vi "Configure Frequency.vi"(0 "VISA resource name":refnum<visa-resource-name>, 5 "Frequency Mode (0: Fixed)":i32(ring) items=["Fixed", "Step", "Pulse", "List", "Sense", "External"], 7 "Frequency (60 Hz)":dbl=60.0, 9 "Triggered Frequency (60 Hz)":dbl=60.0, 11 "error in (no error)":errorcluster) -> (4 "VISA resource name out":refnum<visa-resource-name>, 15 "error out":errorcluster)   [LabVIEW 2013, in "California Instruments iX Series.lvlib"]
doc: "Configures the output frequency of the AC source."
uses:
  California Instruments iX Series.lvlib
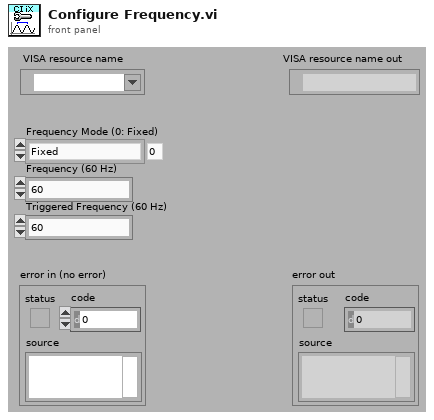
[diagram p1: front panel]
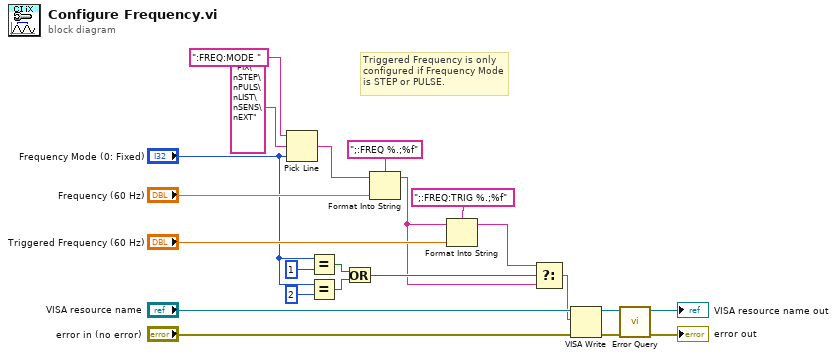
[diagram p0: block diagram]
diagram:
  # "Triggered Frequency is only configured if Frequency Mode is STEP or PULSE."
  n1 = Pick Line(string ("")=":FREQ:MODE ", multi-line string="FIX\nSTEP\nPULS\nLIST\nSENS\nEXT", line index="Frequency Mode (0: Fixed)") -> (output string=w14:string)
  n2 = Equal?(x="Frequency Mode (0: Fixed)", y=1) -> (x = y?=w6:bool)
  n3 = Equal?(x="Frequency Mode (0: Fixed)", y=2) -> (x = y?=w5:bool)
  n4 = Or(x=w6, y=w5) -> (x .or. y?=w4:bool)
  n5 = Format Into String(format string=";:FREQ %.;%f", initial string=w14, "Frequency (60 Hz)") -> (resulting string=w2:string)  [unwired: 1 in, 1 out]
  n6 = Format Into String(format string=";:FREQ:TRIG %.;%f", initial string=w2, "Triggered Frequency (60 Hz)") -> (resulting string=w1:string)  [unwired: 1 in, 1 out]
  n7 = Select(t=w1, s=w4, f=w2) -> (s? t:f=w3:string)
  n8 = VISA Write(VISA resource name="VISA resource name", write buffer=w3, error in (no error)="error in (no error)") -> (VISA resource name out=w18:refnum<visa-resource-name>, error out=w21:errorcluster)  [unwired: 1 out]
  n9 = call "Error Query.vi"("error in (no error)"=w21, "VISA resource name"=w18) -> ("error out"=→"error out":errorcluster, "VISA resource name out"=→"VISA resource name out":refnum<visa-resource-name>)  [unwired: 6 in, 2 out]
